vi "Prepare Control.vi"(7 "VolatusAPI":refnum<class "VolatusAPI.lvclass">, 8 "error in (no error)":errorcluster, 11 "ValveControl in":refnum<class "BangBangControl.lvclass">) -> (0 "error out":errorcluster, 3 "ValveControl out":refnum<class "BangBangControl.lvclass">)   [LabVIEW 2020, in "VolatusControl.lvlib" / "BangBangControl.lvclass"]
uses:
  BangBangControl.lvclass
  Volatus/VolatusAPI/VolatusAPI.lvclass
  BangBangControl.lvclass/BangBangControl.ctl
  Volatus/Module Identity/Module Identity.lvclass/Module Identity.ctl
  lv-vecto/Vecto/Group DBL/Group DBL.lvclass
  C:/dev/lv20CE/relink/lv-vecto/Vecto/Group/Group.lvclass
  Volatus/Module Identity/Create.vi
  Volatus/Module Identity/Module Identity.lvclass
  C:/dev/lv20CE/relink/lv-volatus/Volatus/Identity/Identity.lvclass
  Volatus/VolatusAPI/Lookup Q.vi
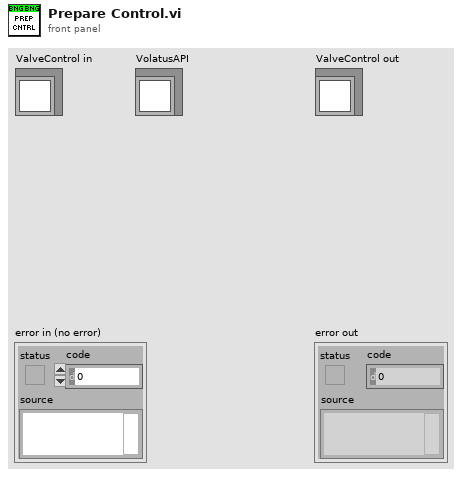
[diagram p1: front panel]
types:
  T1 = typedef "VectoConfig.lvlib/Channel Info.ctl" = cluster{"Name":string, "Group":string, "Owning Node":string, "Owning Task":string, "Resource":string}
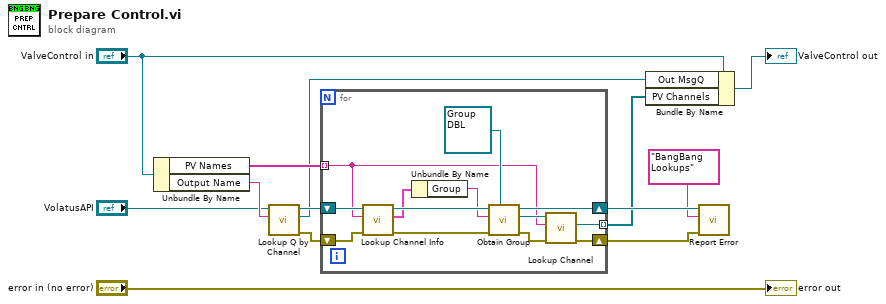
[diagram p0: block diagram]
diagram:
  n1 = Unbundle By Name("ValveControl in") -> ("PV Names"=w7:string[], "Output Name"=w12:string)
  n2 = call "Lookup Q by Channel.vi"("Channel Name"=w12, "VolatusAPI in"="VolatusAPI") -> ("error out"=w10:errorcluster, "MessageQ"=w4:refnum<class "MessageQ.lvclass">, "VolatusAPI out"=w11:refnum<class "VolatusAPI.lvclass">)  [unwired: 7 in]
  n3 = for {
    tunnel: w7 -> [w17] mode=indexing
    tunnel: [w14] -> w5 mode=indexing
    shift-right: [w19] -> w9
    shift-left: w11 -> [w26]
    shift-right: [w15] -> w6
    shift-left: w10 -> [w22]
    n4 = call "Lookup Channel Info.vi"("error in (no error)"=w22, "Channel Name"=w17, "VolatusAPI in"=w26) -> ("error out"=w21:errorcluster, "Channel Info"=w20:T1, "VolatusAPI out"=w25:refnum<class "VolatusAPI.lvclass">)  [unwired: 5 in, 1 out]
    n5 = Unbundle By Name(w20) -> ("Group"=w24:string)
    n6 = call "Obtain Group.vi"("Group Type (Abstract)"=refnum<class "Group DBL.lvclass"> refnum ("Vecto.lvlib:Group.lvclass"), "error in (no error)"=w21, "Group Name"=w24, "VolatusAPI in"=w25) -> ("error out"=w16:errorcluster, "Group"=w18:refnum<class "Group DBL.lvclass">, "VolatusAPI out"=w19:refnum<class "VolatusAPI.lvclass">)  [unwired: 5 in]
    n7 = call "Lookup Channel.vi"("error in (no error)"=w16, "Channel Name"=w17, "Group in"=w18) -> ("error out"=w15:errorcluster, "Channel"=w14:refnum<class "Channel DBL.lvclass">)  [unwired: 6 in, 1 out]
  }
  n8 = Bundle By Name(cluster="ValveControl in", "Out MsgQ"=w4, "PV Channels"=w5) -> (→"ValveControl out":refnum<class "BangBangControl.lvclass">)
  n9 = call "Report Error.vi"("error in (no error)"=w6, "Context"="BangBang Lookups", "VolatusAPI in"=w9) -> ()  [unwired: 7 in, 2 out]
  "error out" <- "error in (no error)"
